vi "helper-log-log.vi"(8 "error in":errorcluster, 10 "ARGS":string, 11 "Enum":T1) -> (0 "error out":errorcluster, 3 "Collected Reports":string)   [LabVIEW 2024]
uses:
  controls/state-logger.ctl
  controls/enum.report-filter.ctl
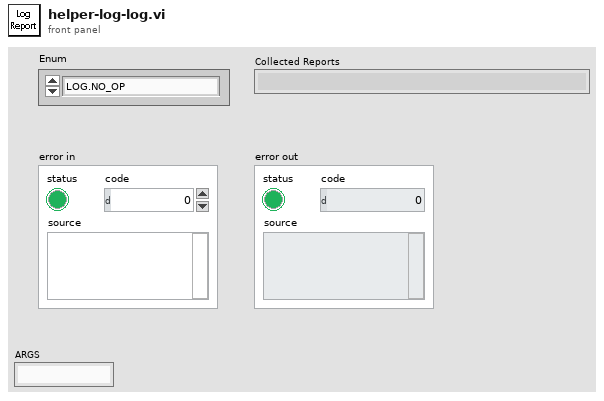
[diagram p1: front panel]
types:
  T1 = typedef "state-logger.ctl" = enum16{"LOG.NO_OP", "LOG.INIT", "LOG.INIT.NTR-FLOW", "LOG.EXIT", "LOG.CATCH", "LOG.PARSE.OCS", "LOG.UPDATE.SELECTORS", "LOG.UPDATE.IRR", "LOG.SNAPSHOT.PROC", "LOG.SNAPSHOT"}
  T2 = typedef "enum.report-filter.ctl" = enum16{"Read ALL", "Read Errors", "Collect", "ClearAll"}
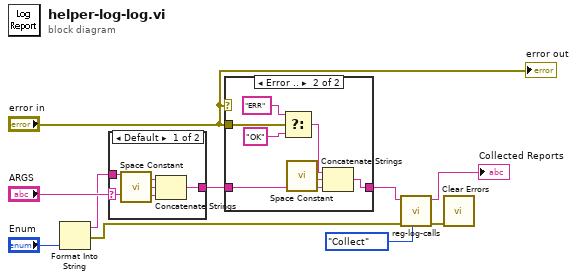
[diagram p0: block diagram]
diagram:
  n1 = Format Into String("Enum") -> (resulting string=w6:string, error out=w4:errorcluster)  [unwired: 3 in]
  n2 = case shown="Default" "ARGS" {
    selector: "ARGS" -> [w12 _]
    tunnel: [w11 w15] -> w3
    tunnel: w6 -> [w14 w15]
    frame Default {
      n3 = call <vilib>:"Space Constant.vi"() -> ("String"=w13:string)
      n4 = Concatenate Strings(w14, w13, w12) -> (w11:string)
    }
    frame "" {
    }
  }
  n5 = case shown="Error .." "error in" {
    tunnel: "error in" -> [_ w23]
    tunnel: w3 -> [w16 w17]
    tunnel: [w16 w21] -> w2
    frame No Error {
    }
    frame Error {
      n6 = Select(t="ERR" ("String"), s=w23, f="OK" ("String")) -> (s? t:f=w18:string)
      n7 = call <vilib>:"Space Constant.vi"() -> ("String"=w22:string)
      n8 = Concatenate Strings(w18, w22, w17) -> (w21:string)
    }
  }
  n9 = call "reg-log-calls.vi"("Operation(Read)"=enum.report-filter."Collect", "error in"=w4, "Reports to Collect"=w2) -> ("error out"=w5:errorcluster, "Collected Reports"=→"Collected Reports":string)  [unwired: 7 in]
  n10 = call <vilib>:"Clear Errors.vi"("error in (no error)"=w5) -> ()  [unwired: 5 in, 2 out]
  "error out" <- "error in"
